vi "Bronkhorst FLOW-BUS Instrument Control Application.vi"() -> ()   [LabVIEW 2024]
doc: "This is the Control Application provided with the Bronkhorst Driver for FLOW-BUS Instruments. The application gives access to the various functions included in the driver. It can be used to test the communication and to control an instrument or as an example to get started with developing your own applications. The basic usage of the application is as follows:\n\n - Start the Application\n - Select the desired COM Port and Baud Rate\n - Click the Connect button\n\nNow data will be collected and saved (if enabled), and commands can be sent to the instrument from the various tab pages. To close the application:\n\n - Open the Setting tab\n - Click Disconnect\n - Click the Exit button to stop the application"
uses:
  <vilib>/Platform/TimedLoop/XDataNode/timing_clust.ctl
  <vilib>/Platform/TimedLoop/XDataNode/nitl_modes.ctl
  <vilib>/Platform/TimedLoop/XDataNode/wakeup.ctl
  <vilib>/Utility/error.llb/DialogType.ctl
  <vilib>/Utility/file.llb/Write To Spreadsheet File (string).vi
  <vilib>/Utility/file.llb/Write To Spreadsheet File (DBL).vi
  <vilib>/Platform/TimedLoop/XDataNode/XDataNode.xnode
  Bronkhorst FLOW-BUS.lvlib
  <vilib>/Platform/TimedLoop/XDataNode/XDNodeRunTimeDep.lvlib
panel:
  in  "Tab Control":T1(tab)=enum."Settings"
  out "Alarm Message":string
  in  "Maximum Limit":dbl=100.0 min=0.0 max=100.0 step=1.0 format="%#g%"
  in  "Minimum Limit":dbl min=0.0 max=100.0 step=1.0 format="%#g%"
  in  "Alarm setpoint mode":u32(ring) items=["No setpoint change at alarm", "Safe setpoint at alarm enabled"]
  in  "Alarm mode":u32(ring) items=["Off", "Alarm on absolute limits", "Alarm on limits related to setpoint (response alarm)", "Alarm when instrument powers up (eg. after power-down)"]
  in  "Alarm Reset Enable":T2={"Keyboard/Micro-Switch"=TRUE, "External"=TRUE, "Reset Parameter"=TRUE, "Automatic"=TRUE}
  in  "Set Alarm Settings":bool
  in  "Alarm Delay Time":u32 format="%.0f Seconds"
  in  "Alarm Setpoint":dbl min=0.0 max=100.0 step=1.0 format="%#g%"
  out "Capacity":sgl
  out "Capacity Unit Display":string
  out "Counter Value":sgl caption="Setpoint %"
  in  "Counter mode":u16(ring) items=["Off", "Counting upwards continuously", "Counting up to limit"]
  in  "Counter setpoint mode":u16(ring) items=["No setpoint change at batch limit allowed", "Setpoint change at batch limit allowed"]
  in  "Counter Setpoint":dbl min=0.0 max=100.0 step=1.0 format="%#g%"
  in  "Counter Limit":sgl min=0 max=1.001638e+07 format="%#.7f"
  in  "Counter Unit":i16(ring)=-1 items=["Select a Unit"=-1, "l"=10, "mm3"=11, "ml"=12, "cm3"=13, "ul"=14, "m3"=15, "g"=20, "mg"=21, "ug"=22, "kg"=23, "ln"=30, "mm3n"=31, "mln"=32, "cm3n"=33, "uln"=34, "dm3n"=35, "m3n"=36, "uls"=37, "mm3s"=38, "mls"=39, "cm3s"=40, "ls"=41, "dm3s"=42, "m3s"=43]
  in  "Set Counter Settings":bool
  in  "Counter Reset Enable":T2={"Keyboard/Micro-Switch"=TRUE, "External"=TRUE, "Reset Parameter"=TRUE, "Automatic"=TRUE}
  in  "Set Fluid Number":bool
  in  "Fluid Number":u8 max=7 step=1
  out "Fluid Name":string
  in  "Reset mode":u16(ring)=5 items=["No Reset", "Reset counter value (no mode change)", "Reset alarm", "Restart batch counter", "Reset counter value (counter off)", "Soft Reset"]
  in  "Reset":bool
  out "Temperature":sgl format="%#_g °C"
  out "Instrument Firmware Revision":string
  out "Analog Input Value":i16 caption="Analog Input"
  out "Instrument Modelnumber":string
  in  "Set Slope":bool
  in  "Setpoint Percentage":dbl min=0.0 max=100.0 step=1.0 format="%#.2g%"
  in  "Setpoint Direct":sgl min=0 step=1 format="%#_g mbar d"
  in  "Seconds":dbl caption="Setpoint Slope" min=0.0 max=3000.0 step=0.1 format="%#.6g Seconds"
  in  "Set Percentage":bool
  in  "Set Direct":bool
  in  "+5":bool
  in  "-5":bool
  in  "-10":bool
  in  "+10":bool
  in  "0":bool
  in  "100":bool
  in  "+1":bool
  in  "-1":bool
  in  "Wink":bool caption="Boolean"
  in  "Connect":bool
  in  "Baud Rate (38400)":u32(ring)=38400 items=["9600"=9600, "19200"=19200, "38400"=38400, "57600"=57600, "115200"=115200, "230400"=230400, "460800"=460800]
  in  "Node Address (3)":u8=3 caption="Node" min=3 max=128 step=1
  in  "Disconnect":bool
  in  "VISA resource name":refnum<visa-resource-name>
  in  "Save Data to File":bool=TRUE
  in  "Stop":bool
  in  "File Location":path
  out "Strip Chart":T3(graph)
  # "(c) 2014 Bronkhorst High-Tech B.V.  ALL RIGHTS RESERVED."
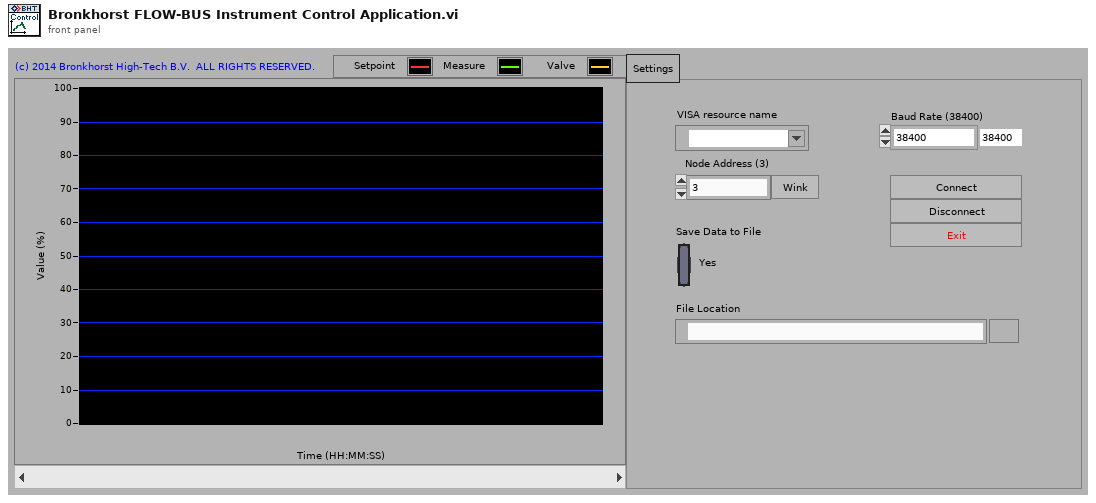
[diagram p1: front panel]
types:
  T1 = enum32{"Alarm", "Capacity", "Counter", "Fluid", "Instrument", "Setpoint", "Settings"}
  T2 = cluster{"Keyboard/Micro-Switch":bool, "External":bool, "Reset Parameter":bool, "Automatic":bool}
  T3 = cluster{"Measure Percentage":dbl, "Setpoint Percentage":dbl, "Valve Output Percentage":dbl}
  T4 = typedef "XDNodeRunTimeDep.lvlib/timing_clust.ctl" = cluster{"Expected End [f-1]":u64, "Actual End [f-1]":u64, "Finished Late? [f-1]":bool, "Expected End [i-1]":u64, "Actual End [i-1]":u64, "Finished Late? [i-1]":bool, "Expected Start [i]":u64, "Actual Start [i]":u64, "Expected Start [f]":u64, "Actual Start [f]":u64, "Source Name":string, "Structure Name":string, "Period":i64, "Deadline":i64, "Offset":i64, "Start":i64, "Priority":i32, "Timeout":i32, "Mode":T5, "Wakeup Reason":T6, "Error":errorcluster, "Source Type":string, "Secondary Source Type":string, "Global End Time":u64, "Global Start Time":u64, "Frame Duration":u64, "Iteration Duration":u64, "Assigned CPU":i32, "I/O Scan Engine Mode":u32}
  T5 = typedef "XDNodeRunTimeDep.lvlib/nitl_modes.ctl" = enum32{"No Change", "Process missed periods, maintain original phase", "Discard missed periods, maintain original phase", "Process missed periods, ignore original phase", "Discard missed periods, ignore original phase"}
  T6 = typedef "XDNodeRunTimeDep.lvlib/wakeup.ctl" = enum32{"Normal", "Aborted", "Asynchronous wakeup", "Timing source error", "Timed loop error", "Timeout"}
  T7 = enum16{"open", "replace", "create", "open or create", "replace or create", "replace or create with confirmation"}
  T8 = typedef "DialogType.ctl" = u16
  T9 = cluster{"Setpoint Percentage":dbl, "Measure Percentage":dbl, "Valve Output Percentage":dbl}
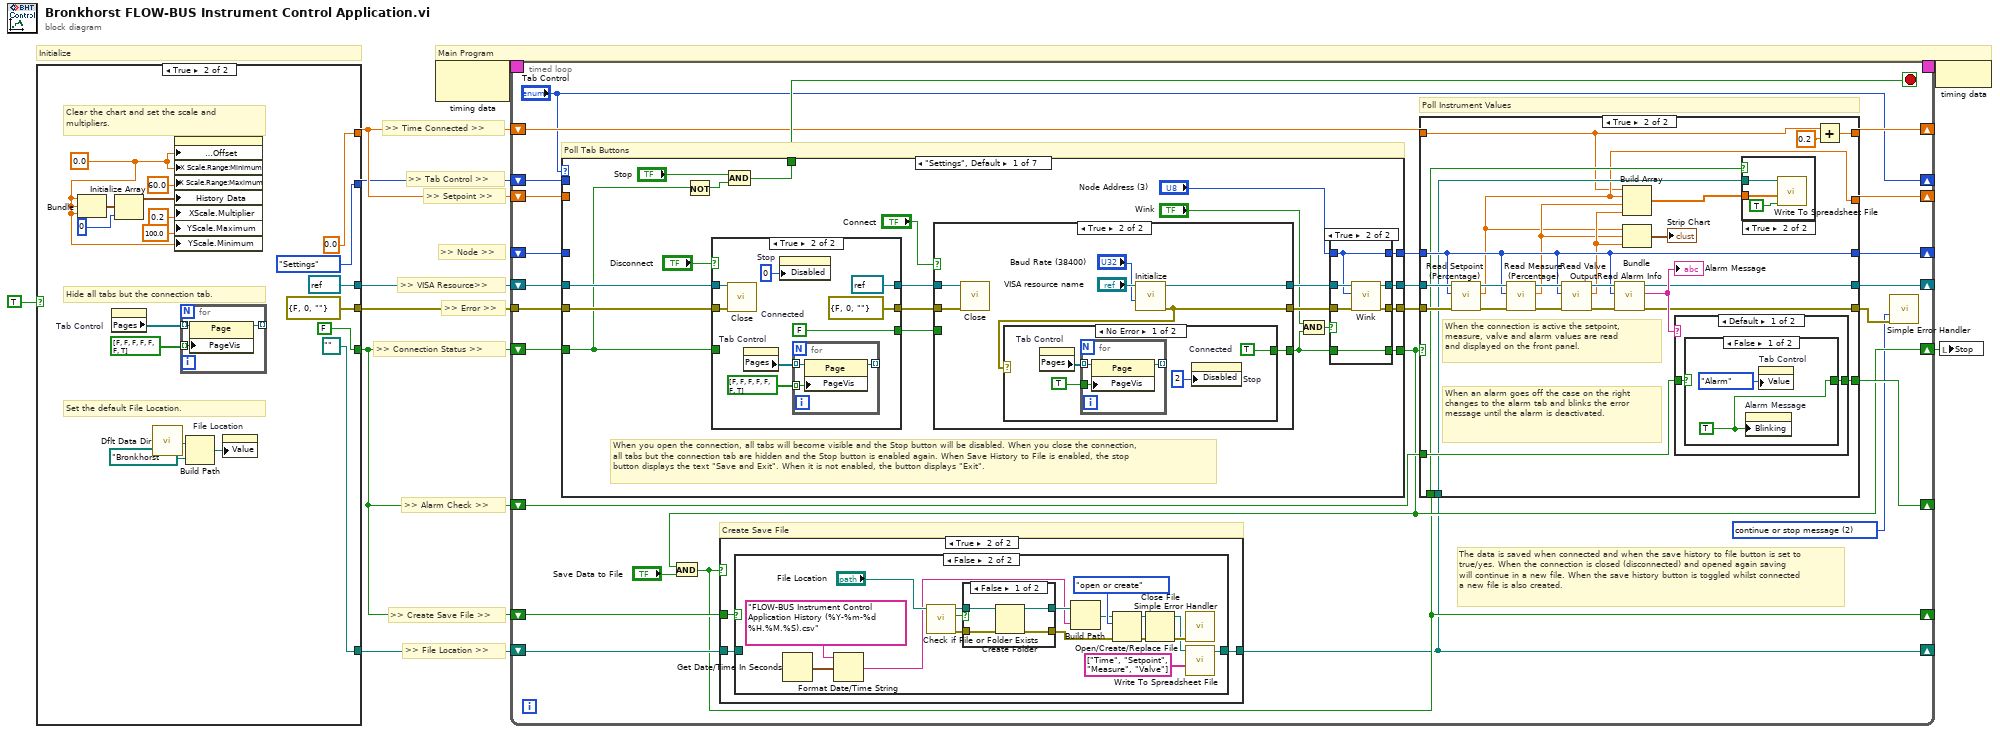
[diagram p0: block diagram]
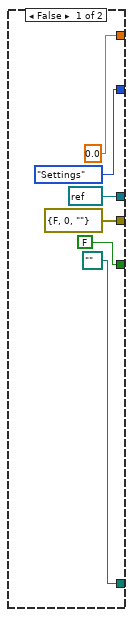
[diagram p2: hidden frame]
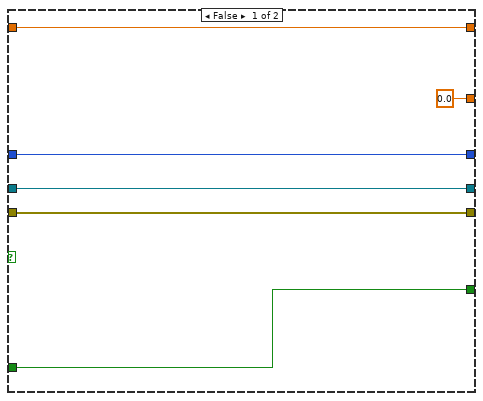
[diagram p6: hidden frame]
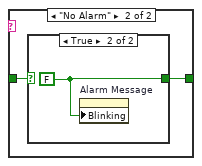
[diagram p9: hidden frame]
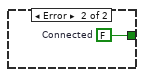
[diagram p14: hidden frame]
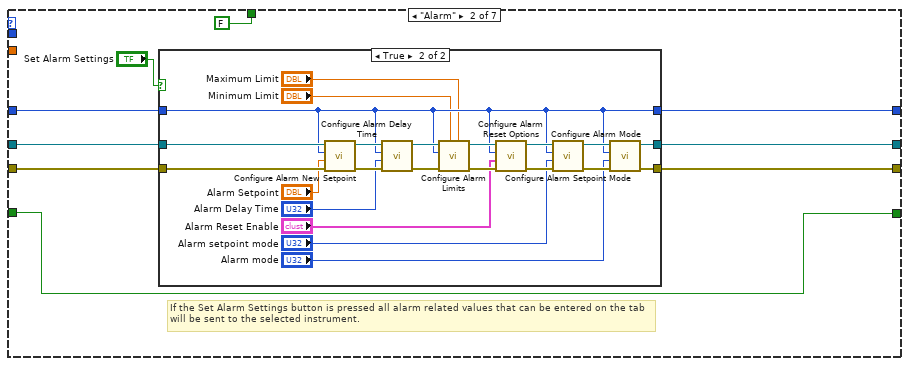
[diagram p15: hidden frame]
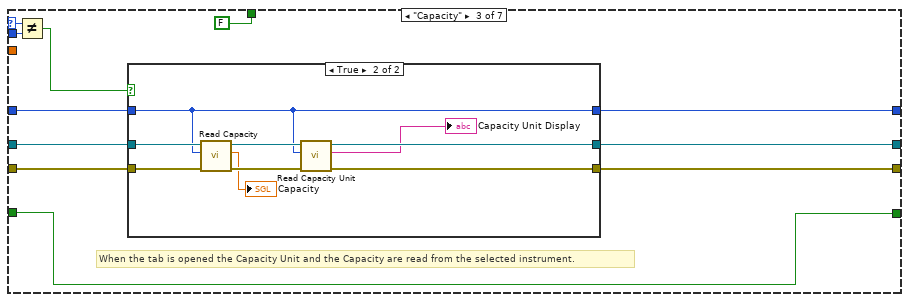
[diagram p17: hidden frame]
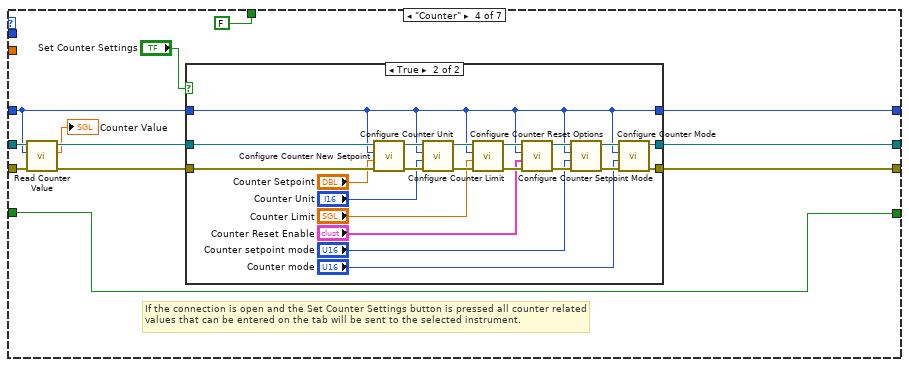
[diagram p19: hidden frame]
diagram:
  # ">> File Location >>"
  # ">> Create Save File >>"
  # "Initialize"
  # "Main Program"
  # ">> Setpoint >>"
  # ">> Time Connected >>"
  # ">> Tab Control >>"
  # ">> Alarm Check >>"
  # ">> Connection Status >>"
  # ">> Node >>"
  # ">> VISA Resource>>"
  # ">> Error >>"
  n1 = case shown="True" TRUE {
    tunnel: [errorcluster {"status"=FALSE, "code"=0, "source"=""} ("error out") errorcluster {"status"=FALSE, "code"=0, "source"=""} ("error out")] -> w1
    tunnel: [refnum<visa-resource-name> refnum ("VISA resource name out") refnum<visa-resource-name> refnum ("VISA resource name out")] -> w8
    tunnel: [T1."Settings" ("Tab Control") T1."Settings" ("Tab Control")] -> w6
    tunnel: [0.0 0.0] -> w7
    tunnel: [FALSE ("Connected") FALSE ("Connected")] -> w4
    tunnel: [path "" ("new file path (Not A Path if cancelled)") path "" ("new file path (Not A Path if cancelled)")] -> w3
    frame False {
    }
    frame True {
      w21 = 0.0
      # "Set the default File Location."
      # "Hide all tabs but the connection tab."
      # "Clear the chart and set the scale and multipliers."
      n2 = Bundle(w21, w21, w21) -> (w30:cluster{dbl, dbl, dbl})  [unwired: 1 in]
      n3 = property on="Tab Control" class="TabCtl (strict)"() -> ("Pages"=w34:refnum<vi>[])  [unwired: 2 in, 2 out]
      n4 = Initialize Array(w30, 0) -> (w32:cluster{dbl, dbl, dbl}[])
      n5 = call <vilib>:"Dflt Data Dir.vi"() -> ("App:Default Data Directory"=w18:path)
      n6 = property on="Strip Chart" class="WFChart (strict)"("X Scale.Offset and Multiplier:Offset"=w21, "X Scale.Range:Minimum"=w21, "X Scale.Range:Maximum"=60.0, "History Data"=w32, "XScale.Multiplier"=0.2 ("y"), "YScale.Maximum"=100.0, "YScale.Minimum"=w21) -> ()  [unwired: 2 in, 2 out]
      n7 = for {
        tunnel: w34 -> [w37] mode=indexing
        tunnel: bool[] [FALSE, FALSE, FALSE, FALSE, FALSE, FALSE, TRUE] -> [w36] mode=indexing
        tunnel: [w35] -> _ mode=indexing
        n8 = property class="Page"(reference=w37, "PageVis"=w36) -> (reference out=w35:refnum<vi>)  [unwired: 1 in, 1 out]
      }
      n9 = Build Path(base path=w18, name or relative path=path "Bronkhorst") -> (appended path=w20:path)
      n10 = property on="File Location" class="Path"("Value"=w20) -> ()  [unwired: 2 in, 2 out]
    }
  }
  n11 = node-c288() -> (w9:T4)  [unwired: 1 in]
  n12 = timed-loop {
    timing-out: [_] -> w10
    timing: w9 -> [_]
    shift-right: [w48] -> w2
    shift-left: w4 -> [w49]
    shift-right: [w41] -> _
    shift-left: w8 -> [w60]
    shift-right: [w42] -> _
    shift-left: _ -> [w61]
    shift-right: [w53] -> _
    shift-left: w7 -> [w62]
    shift-right: [w56] -> _
    shift-left: w4 -> [w55]
    shift-right: ["Tab Control"] -> _
    shift-left: w6 -> [w54]
    shift-right: [w52] -> _
    shift-left: w7 -> [w44]
    shift-right: [w46] -> _
    shift-left: w4 -> [w51]
    shift-right: [w45] -> _
    shift-left: w3 -> [w50]
    tunnel: w1 -> [w39]
    stop <- w63 stop-if-true
    w38 = T8 2 items=["no dialog", "OK message", "continue or stop message", "OK message + warnings", "continue/stop + warnings"] ("type of dialog (OK msg:1)")
    # "Poll Instrument Values"
    # "The data is saved when connected and when the save history to file button is set to true/yes. When the connection is closed (disconnected) and opened again saving will continue in a new file. When the save history button is toggled whilst connected a new file is also created."
    # "Create Save File"
    # "Poll Tab Buttons"
    n13 = case shown="\"Settings\", Default" "Tab Control" {
      selector: "Tab Control" -> [_ _ w237 _ w304 w333 w373]
      tunnel: [w142 w205 w234 w260 w300 w338 w369] -> w58
      tunnel: [w141 w204 w233 w261 w299 w336 w368] -> w57
      tunnel: w60 -> [w153 w203 w239 w256 w302 w328 w372]
      tunnel: w39 -> [w151 w202 w241 w259 w301 w327 w371]
      tunnel: [w136 w200 w232 w263 w296 w341 w370] -> w59
      tunnel: w61 -> [_ w201 w240 w255 w303 w326 w365]
      tunnel: [w137 w197 w235 w265 w291 w335 w375] -> w48
      tunnel: w49 -> [w144 w197 w235 w265 w291 w335 w375]
      tunnel: w62 -> [_ _ _ _ _ _ w367]
      tunnel: w54 -> [_ _ w238 _ w305 w334 w374]
      tunnel: [w146 FALSE ("stop") FALSE ("stop") FALSE ("stop") FALSE ("stop") FALSE ("stop") FALSE ("stop")] -> w63
      frame "Settings", Default {
        # "When you open the connection, all tabs will become visible and the Stop button will be disabled. When you close the connection, all tabs but the connection tab are hidden and the Stop button is enabled again. When Save History to File is enabled, the stop button displays the text \"Save and Exit\". When it is not enabled, the button displays \"Exit\"."
        n14 = Not(x=w144) -> (.not. x?=w147:bool)
        n15 = case shown="True" "Disconnect" {
          tunnel: w153 -> [w167 w172]
          tunnel: [w167 refnum<visa-resource-name> refnum ("VISA resource name out")] -> w152
          tunnel: [w166 errorcluster {"status"=FALSE, "code"=0, "source"=""} ("error out")] -> w150
          tunnel: w151 -> [w166 w171]
          tunnel: [w165 w175] -> w148
          tunnel: w144 -> [w165 _]
          frame False {
          }
          frame True {
            w175 = FALSE  # Connected
            n16 = call "Close.vi"("error in (no error)"=w171, "VISA resource name"=w172) -> ()  [unwired: 9 in, 1 out]
            n17 = property on="Tab Control" class="TabCtl (strict)"() -> ("Pages"=w173:refnum<vi>[])  [unwired: 2 in, 2 out]
            n18 = property on="Stop" class="Bool (strict)"("Disabled"=u8 0) -> ()  [unwired: 2 in, 2 out]
            n19 = for {
              tunnel: w173 -> [w178] mode=indexing
              tunnel: [w177] -> _ mode=indexing
              tunnel: bool[] [FALSE, FALSE, FALSE, FALSE, FALSE, FALSE, TRUE] -> [w176] mode=indexing
              n20 = property class="Page"(reference=w178, "PageVis"=w176) -> (reference out=w177:refnum<vi>)  [unwired: 1 in, 1 out]
            }
          }
        }
        n21 = And(x="Stop", y=w147) -> (x .and. y?=w146:bool)
        n22 = case shown="True" "Connect" {
          tunnel: [w180 w183] -> w140
          tunnel: [w181 w182] -> w139
          tunnel: w152 -> [w180 w185]
          tunnel: w150 -> [w181 w186]
          tunnel: [w179 w184] -> w134
          tunnel: w148 -> [w179 _]
          frame False {
          }
          frame True {
            n23 = call "Close.vi"("error in (no error)"=w186, "VISA resource name"=w185) -> ()  [unwired: 9 in, 1 out]
            n24 = call "Initialize.vi"("Baud Rate (38400)"="Baud Rate (38400)", "VISA resource name"="VISA resource name") -> ("error out"=w182:errorcluster, "VISA resource name out"=w183:refnum<visa-resource-name>)  [unwired: 8 in]
            n25 = case shown="No Error" w182 {
              tunnel: [w189 w196] -> w184
              frame No Error {
                w189 = TRUE  # Connected
                n26 = property on="Tab Control" class="TabCtl (strict)"() -> ("Pages"=w191:refnum<vi>[])  [unwired: 2 in, 2 out]
                n27 = for {
                  tunnel: w191 -> [w195] mode=indexing
                  tunnel: TRUE -> [w194]
                  tunnel: [w193] -> _ mode=indexing
                  n28 = property class="Page"(reference=w195, "PageVis"=w194) -> (reference out=w193:refnum<vi>)  [unwired: 1 in, 1 out]
                }
                n29 = property on="Stop" class="Bool (strict)"("Disabled"=u8 2) -> ()  [unwired: 2 in, 2 out]
              }
              frame Error {
                w196 = FALSE  # Connected
              }
            }
          }
        }
        n30 = And(x="Wink", y=w134) -> (x .and. y?=w138:bool)
        n31 = case shown="True" w138 {
          tunnel: "Node Address (3)" -> [w155 w159]
          tunnel: [w158 w164] -> w142
          tunnel: [w157 w163] -> w141
          tunnel: w140 -> [w158 w161]
          tunnel: w139 -> [w157 w162]
          tunnel: [w156 w160] -> w137
          tunnel: w134 -> [w156 w160]
          tunnel: [w155 w159] -> w136
          frame False {
          }
          frame True {
            n32 = call "Wink.vi"("error in (no error)"=w162, "Node (3)"=w159, "VISA resource name"=w161) -> ("error out"=w163:errorcluster, "VISA resource name out"=w164:refnum<visa-resource-name>)  [unwired: 7 in]
          }
        }
      }
      frame "Alarm" {
        # "If the Set Alarm Settings button is pressed all alarm related values that can be entered on the tab will be sent to the selected instrument."
        n33 = case shown="True" "Set Alarm Settings" {
          tunnel: w203 -> [w207 w230]
          tunnel: w202 -> [w206 w229]
          tunnel: w201 -> [w208 w213]
          tunnel: [w207 w223] -> w205
          tunnel: [w206 w222] -> w204
          tunnel: [w208 w213] -> w200
          frame False {
          }
          frame True {
            n34 = call "Configure Alarm New Setpoint.vi"("error in (no error)"=w229, "Alarm Setpoint (0%)"="Alarm Setpoint", "Node (3)"=w213, "VISA resource name"=w230) -> ("error out"=w227:errorcluster, "VISA resource name out"=w228:refnum<visa-resource-name>)  [unwired: 6 in]
            n35 = call "Configure Alarm Delay Time.vi"("error in (no error)"=w227, "Alarm Delay Time (0 Seconds)"="Alarm Delay Time", "Node (3)"=w213, "VISA resource name"=w228) -> ("error out"=w214:errorcluster, "VISA resource name out"=w217:refnum<visa-resource-name>)  [unwired: 6 in]
            n36 = call "Configure Alarm Limits.vi"("Maximum Limit (100%)"="Maximum Limit", "Minimum Limit (0%)"="Minimum Limit", "error in (no error)"=w214, "Node (3)"=w213, "VISA resource name"=w217) -> ("error out"=w215:errorcluster, "VISA resource name out"=w216:refnum<visa-resource-name>)  [unwired: 5 in]
            n37 = call "Configure Alarm Reset Options.vi"("error in (no error)"=w215, "Alarm Reset (All Enabled)"="Alarm Reset Enable", "Node (3)"=w213, "VISA resource name"=w216) -> ("error out"=w224:errorcluster, "VISA resource name out"=w225:refnum<visa-resource-name>)  [unwired: 6 in]
            n38 = call "Configure Alarm Setpoint Mode.vi"("error in (no error)"=w224, "Alarm Setpoint Mode (0: No setpoint)"="Alarm setpoint mode", "Node (3)"=w213, "VISA resource name"=w225) -> ("error out"=w221:errorcluster, "VISA resource name out"=w220:refnum<visa-resource-name>)  [unwired: 6 in]
            n39 = call "Configure Alarm Mode.vi"("error in (no error)"=w221, "Alarm mode (0: Off)"="Alarm mode", "Node (3)"=w213, "VISA resource name"=w220) -> ("error out"=w222:errorcluster, "VISA resource name out"=w223:refnum<visa-resource-name>)  [unwired: 6 in]
          }
        }
      }
      frame "Capacity" {
        # "When the tab is opened the Capacity Unit and the Capacity are read from the selected instrument."
        n40 = Not Equal?(x=w237, y=w238) -> (x != y?=w231:bool)
        n41 = case shown="True" w231 {
          tunnel: w239 -> [w243 w253]
          tunnel: w241 -> [w242 w252]
          tunnel: w240 -> [w244 w246]
          tunnel: [w243 w248] -> w234
          tunnel: [w242 w249] -> w233
          tunnel: [w244 w246] -> w232
          frame False {
          }
          frame True {
            n42 = call "Read Capacity.vi"("error in (no error)"=w252, "Node (3)"=w246, "VISA resource name"=w253) -> ("error out"=w250:errorcluster, "Capacity"=→"Capacity":sgl, "VISA resource name out"=w251:refnum<visa-resource-name>)  [unwired: 6 in]
            n43 = call "Read Capacity Unit.vi"("error in (no error)"=w250, "Node (3)"=w246, "VISA resource name"=w251) -> ("error out"=w249:errorcluster, "Capacity Unit"=→"Capacity Unit Display":string, "VISA resource name out"=w248:refnum<visa-resource-name>)  [unwired: 6 in]
          }
        }
      }
      frame "Counter" {
        # "If the connection is open and the Set Counter Settings button is pressed all counter related values that can be entered on the tab will be sent to the selected instrument."
        n44 = call "Read Counter Value.vi"("error in (no error)"=w259, "Node (3)"=w255, "VISA resource name"=w256) -> ("error out"=w258:errorcluster, "Counter Value"=→"Counter Value":sgl, "VISA resource name out"=w257:refnum<visa-resource-name>)  [unwired: 6 in]
        n45 = case shown="True" "Set Counter Settings" {
          tunnel: w257 -> [w267 w274]
          tunnel: w258 -> [w266 w273]
          tunnel: w255 -> [w268 w269]
          tunnel: [w267 w272] -> w260
          tunnel: [w266 w271] -> w261
          tunnel: [w268 w269] -> w263
          frame False {
          }
          frame True {
            n46 = call "Configure Counter New Setpoint.vi"("error in (no error)"=w273, "Counter Setpoint (0%)"="Counter Setpoint", "Node (3)"=w269, "VISA resource name"=w274) -> ("error out"=w280:errorcluster, "VISA resource name out"=w289:refnum<visa-resource-name>)  [unwired: 6 in]
            n47 = call "Configure Counter Unit.vi"("error in (no error)"=w280, "Counter Unit (-1:Select a Unit)"="Counter Unit", "Node (3)"=w269, "VISA resource name"=w289) -> ("error out"=w281:errorcluster, "VISA resource name out"=w288:refnum<visa-resource-name>)  [unwired: 6 in]
            n48 = call "Configure Counter Limit.vi"("error in (no error)"=w281, "Counter Limit (0)"="Counter Limit", "Node (3)"=w269, "VISA resource name"=w288) -> ("error out"=w282:errorcluster, "VISA resource name out"=w287:refnum<visa-resource-name>)  [unwired: 6 in]
            n49 = call "Configure Counter Reset Options.vi"("error in (no error)"=w282, "Counter Reset (All Enabled)"="Counter Reset Enable", "Node (3)"=w269, "VISA resource name"=w287) -> ("error out"=w283:errorcluster, "VISA resource name out"=w286:refnum<visa-resource-name>)  [unwired: 6 in]
            n50 = call "Configure Counter Setpoint Mode.vi"("error in (no error)"=w283, "Counter setpoint mode (0: No setpoint change)"="Counter setpoint mode", "Node (3)"=w269, "VISA resource name"=w286) -> ("error out"=w284:errorcluster, "VISA resource name out"=w285:refnum<visa-resource-name>)  [unwired: 6 in]
            n51 = call "Configure Counter Mode.vi"("error in (no error)"=w284, "Counter Mode (0: Off)"="Counter mode", "Node (3)"=w269, "VISA resource name"=w285) -> ("error out"=w271:errorcluster, "VISA resource name out"=w272:refnum<visa-resource-name>)  [unwired: 6 in]
          }
        }
      }
      frame "Fluid" {
        # "If the connection is open and the Set Fluid Number button is pressed, the selected fluid number will be sent to, and the fluid name will be read from the selected instrument. When the tab is opened the Fluid name will be read from the selected instrument."
        n52 = Not Equal?(x=w304, y=w305) -> (x != y?=w292:bool)
        n53 = case shown="True" "Set Fluid Number" {
          tunnel: [w317 w319] -> w295
          tunnel: w303 -> [w317 w319]
          tunnel: w302 -> [w316 w323]
          tunnel: w301 -> [w315 w322]
          tunnel: [w316 w321] -> w297
          tunnel: [w315 w320] -> w298
          frame False {
          }
          frame True {
            n54 = call "Configure Fluid Number.vi"("error in (no error)"=w322, "Fluid Number (0)"="Fluid Number", "Node (3)"=w319, "VISA resource name"=w323) -> ("error out"=w320:errorcluster, "VISA resource name out"=w321:refnum<visa-resource-name>)  [unwired: 6 in]
          }
        }
        n55 = Or(x=w292, y="Set Fluid Number") -> (x .or. y?=w294:bool)
        n56 = case shown="True" w294 {
          tunnel: [w307 w314] -> w300
          tunnel: [w306 w313] -> w299
          tunnel: w298 -> [w306 w312]
          tunnel: w297 -> [w307 w311]
          tunnel: [w308 w310] -> w296
          tunnel: w295 -> [w308 w310]
          frame False {
          }
          frame True {
            n57 = call "Read Fluid Name.vi"("error in (no error)"=w312, "Node (3)"=w310, "VISA resource name"=w311) -> ("error out"=w313:errorcluster, "Fluid Name"=→"Fluid Name":string, "VISA resource name out"=w314:refnum<visa-resource-name>)  [unwired: 6 in]
          }
        }
      }
      frame "Instrument" {
        # "When the tab is opened, all values on the tab will be read from the selected instrument. When the connection is active and the reset button is pressed, the selected reset command will be sent to the selected instrument."
        n58 = Not Equal?(x=w333, y=w334) -> (x != y?=w332:bool)
        n59 = call "Read Analog Input.vi"("error in (no error)"=w327, "Node (3)"=w326, "VISA resource name"=w328) -> ("error out"=w330:errorcluster, "Analog Input Value"=→"Analog Input Value":i16, "VISA resource name out"=w329:refnum<visa-resource-name>)  [unwired: 6 in]
        n60 = case shown="True" w332 {
          tunnel: w329 -> [w352 w359]
          tunnel: w330 -> [w351 w360]
          tunnel: w326 -> [w353 w357]
          tunnel: [w352 w363] -> w339
          tunnel: [w351 w362] -> w337
          tunnel: [w353 w357] -> w340
          frame False {
          }
          frame True {
            n61 = call "Read Temperature.vi"("error in (no error)"=w360, "Node (3)"=w357, "VISA resource name"=w359) -> ("error out"=w356:errorcluster, "Temperature (deg C)"=→"Temperature":sgl, "VISA resource name out"=w355:refnum<visa-resource-name>)  [unwired: 6 in]
            n62 = call "Revision Query.vi"("error in (no error)"=w356, "Node (3)"=w357, "VISA resource name"=w355) -> ("error out"=w362:errorcluster, "Instrument Firmware Revision"=→"Instrument Firmware Revision":string, "VISA resource name out"=w363:refnum<visa-resource-name>, "Instrument Modelnumber"=→"Instrument Modelnumber":string)  [unwired: 4 in, 1 out]
          }
        }
        n63 = case shown="True" "Reset" {
          tunnel: w340 -> [w344 w348]
          tunnel: [w344 w348] -> w341
          tunnel: w339 -> [w343 w350]
          tunnel: [w343 w346] -> w338
          tunnel: [w342 w345] -> w336
          tunnel: w337 -> [w342 w349]
          frame False {
          }
          frame True {
            n64 = call "Reset.vi"("error in (no error)"=w349, "Reset mode (5: Soft Reset)"="Reset mode", "Node (3)"=w348, "VISA resource name"=w350) -> ("error out"=w345:errorcluster, "VISA resource name out"=w346:refnum<visa-resource-name>)  [unwired: 6 in]
          }
        }
      }
      frame "Setpoint" {
        # "When the tab is opened the setpoint is read from the instrument (both percentage and direct) and displayed in the indicators. When any of the buttons are pressed the corresponding action is performed."
        n65 = Not Equal?(x=w373, y=w374) -> (x != y?=w364:bool)
        n66 = case shown="True" w364 {
          tunnel: [w390 w504] -> w370
          tunnel: w365 -> [w395 w504]
          tunnel: w372 -> [w393 w511]
          tunnel: w371 -> [w394 w510]
          tunnel: [w389 w502] -> w368
          tunnel: [w392 w503] -> w369
          tunnel: w367 -> [w391 _]
          frame False {
            # "The booleans are turned into a number so multiple buttons can be checked in one case."
            n67 = Build Array("-5", "+5", "-10", "+10", "0", "100", "-1", "+1") -> (w384:bool[])
            n68 = Boolean Array To Number(Boolean array=w384) -> (number=w388:u32)
            n69 = case shown="1" w388 {
              tunnel: [w408 w421 w429 w437 w443 w449 w457 w465 w470] -> w405
              tunnel: w395 -> [w408 w421 w429 w437 w443 w449 w457 w465 w470]
              tunnel: [w415 w423 w431 w439 w445 w451 w459 w467 w469] -> w406
              tunnel: w393 -> [w413 w420 w428 w436 w442 w448 w456 w464 w469]
              tunnel: w394 -> [w412 w419 w427 w435 w441 w447 w455 w463 w468]
              tunnel: [w414 w422 w430 w438 w444 w450 w458 w466 w468] -> w407
              tunnel: w391 -> [w410 w417 w425 w433 _ _ w453 w461 _]
              frame 1 {
                n70 = Subtract(x=w410, y=5.0) -> (x-y=w409:dbl)
                n71 = call "Configure Setpoint (Percentage).vi"("error in (no error)"=w412, "Setpoint Percentage (0%)"=w409, "Node (3)"=w408, "VISA resource name"=w413) -> ("error out"=w414:errorcluster, "VISA resource name out"=w415:refnum<visa-resource-name>)  [unwired: 6 in]
              }
              frame 2 {
                n72 = Add(x=w417, y=5.0) -> (x+y=w416:dbl)
                n73 = call "Configure Setpoint (Percentage).vi"("error in (no error)"=w419, "Setpoint Percentage (0%)"=w416, "Node (3)"=w421, "VISA resource name"=w420) -> ("error out"=w422:errorcluster, "VISA resource name out"=w423:refnum<visa-resource-name>)  [unwired: 6 in]
              }
              frame 4 {
                n74 = Subtract(x=w425, y=10.0) -> (x-y=w424:dbl)
                n75 = call "Configure Setpoint (Percentage).vi"("error in (no error)"=w427, "Setpoint Percentage (0%)"=w424, "Node (3)"=w429, "VISA resource name"=w428) -> ("error out"=w430:errorcluster, "VISA resource name out"=w431:refnum<visa-resource-name>)  [unwired: 6 in]
              }
              frame 8 {
                n76 = Add(x=w433, y=10.0) -> (x+y=w432:dbl)
                n77 = call "Configure Setpoint (Percentage).vi"("error in (no error)"=w435, "Setpoint Percentage (0%)"=w432, "Node (3)"=w437, "VISA resource name"=w436) -> ("error out"=w438:errorcluster, "VISA resource name out"=w439:refnum<visa-resource-name>)  [unwired: 6 in]
              }
              frame 16 {
                n78 = call "Configure Setpoint (Percentage).vi"("error in (no error)"=w441, "Setpoint Percentage (0%)"=0.0 ("y"), "Node (3)"=w443, "VISA resource name"=w442) -> ("error out"=w444:errorcluster, "VISA resource name out"=w445:refnum<visa-resource-name>)  [unwired: 6 in]
              }
              frame 32 {
                n79 = call "Configure Setpoint (Percentage).vi"("error in (no error)"=w447, "Setpoint Percentage (0%)"=100.0 ("y"), "Node (3)"=w449, "VISA resource name"=w448) -> ("error out"=w450:errorcluster, "VISA resource name out"=w451:refnum<visa-resource-name>)  [unwired: 6 in]
              }
              frame 64 {
                n80 = Subtract(x=w453, y=1.0) -> (x-y=w452:dbl)
                n81 = call "Configure Setpoint (Percentage).vi"("error in (no error)"=w455, "Setpoint Percentage (0%)"=w452, "Node (3)"=w457, "VISA resource name"=w456) -> ("error out"=w458:errorcluster, "VISA resource name out"=w459:refnum<visa-resource-name>)  [unwired: 6 in]
              }
              frame 128 {
                n82 = Add(x=w461, y=1.0) -> (x+y=w460:dbl)
                n83 = call "Configure Setpoint (Percentage).vi"("error in (no error)"=w463, "Setpoint Percentage (0%)"=w460, "Node (3)"=w465, "VISA resource name"=w464) -> ("error out"=w466:errorcluster, "VISA resource name out"=w467:refnum<visa-resource-name>)  [unwired: 6 in]
              }
              frame Default {
              }
            }
            n84 = case shown="True" "Set Slope" {
              tunnel: [w471 w474] -> w400
              tunnel: [w472 w475] -> w401
              tunnel: [w473 w478] -> w403
              tunnel: w405 -> [w473 w478]
              tunnel: w407 -> [w472 w477]
              tunnel: "Seconds" -> [_ w476]
              tunnel: w406 -> [w471 w479]
              frame False {
              }
              frame True {
                n85 = call "Configure Setpoint Slope.vi"("error in (no error)"=w477, "Setpoint Slope (0 Seconds)"=w476, "Node (3)"=w478, "VISA resource name"=w479) -> ("error out"=w475:errorcluster, "VISA resource name out"=w474:refnum<visa-resource-name>)  [unwired: 6 in]
              }
            }
            n86 = case shown="True" "Set Percentage" {
              tunnel: [w491 w495] -> w399
              tunnel: [w490 w494] -> w398
              tunnel: w400 -> [w491 w497]
              tunnel: w401 -> [w490 w496]
              tunnel: "Setpoint Percentage" -> [_ w492]
              tunnel: w403 -> [w489 w493]
              tunnel: [w489 w493] -> w404
              frame False {
              }
              frame True {
                n87 = call "Configure Setpoint (Percentage).vi"("error in (no error)"=w496, "Setpoint Percentage (0%)"=w492, "Node (3)"=w493, "VISA resource name"=w497) -> ("error out"=w494:errorcluster, "VISA resource name out"=w495:refnum<visa-resource-name>)  [unwired: 6 in]
              }
            }
            n88 = case shown="True" "Set Direct" {
              tunnel: [w481 w486] -> w392
              tunnel: [w482 w485] -> w389
              tunnel: w399 -> [w481 w488]
              tunnel: w398 -> [w482 w487]
              tunnel: "Setpoint Direct" -> [_ w484]
              tunnel: [w480 w483] -> w390
              tunnel: w404 -> [w480 w483]
              frame False {
              }
              frame True {
                n89 = call "Configure Setpoint (Direct).vi"("error in (no error)"=w487, "Setpoint Direct (0)"=w484, "Node (3)"=w483, "VISA resource name"=w488) -> ("error out"=w485:errorcluster, "VISA resource name out"=w486:refnum<visa-resource-name>)  [unwired: 6 in]
              }
            }
          }
          frame True {
            n90 = call "Read Setpoint (Percentage).vi"("error in (no error)"=w510, "Node (3)"=w504, "VISA resource name"=w511) -> ("error out"=w508:errorcluster, "Setpoint Percentage"=w507:dbl, "VISA resource name out"=w509:refnum<visa-resource-name>)  [unwired: 6 in]
            n91 = call "Read Setpoint (Direct).vi"("error in (no error)"=w508, "Node (3)"=w504, "VISA resource name"=w509) -> ("error out"=w506:errorcluster, "Setpoint Direct"=w498:sgl, "VISA resource name out"=w505:refnum<visa-resource-name>)  [unwired: 6 in]
            n92 = call "Read Capacity Unit.vi"("error in (no error)"=w506, "Node (3)"=w504, "VISA resource name"=w505) -> ("error out"=w502:errorcluster, "Capacity Unit"=w499:string, "VISA resource name out"=w503:refnum<visa-resource-name>)  [unwired: 6 in]
            n93 = Concatenate Strings("%#_g ", w499) -> (w501:string)
            n94 = local write "Setpoint Direct"(w498) -> ()
            n95 = local write "Setpoint Percentage"(w507) -> ()
            n96 = property on="Setpoint Direct" class="DigNum (strict)"("FormatString"=w501) -> ()  [unwired: 2 in, 2 out]
          }
        }
      }
    }
    n97 = And(x=w48, y="Save Data to File") -> (x .and. y?=w46:bool)
    n98 = case shown="True" w46 {
      tunnel: [w64 w67] -> w45
      tunnel: w51 -> [_ w66]
      tunnel: w50 -> [w64 w65]
      frame False {
      }
      frame True {
        n99 = case shown="False" w66 {
          tunnel: [w68 w71] -> w67
          tunnel: w65 -> [w68 _]
          frame True {
          }
          frame False {
            n100 = Get Date/Time In Seconds() -> (seconds since 1Jan1904=w73:timestamp)
            n101 = Format Date/Time String(time format string (%c)="FLOW-BUS Instrument Control Application History (%Y-%m-%d %H.%M.%S).csv", seconds (now)=w73) -> (date/time string=w69:string)  [unwired: 1 in]
            n102 = call <vilib>:"Check if File or Folder Exists.vi"("path"="File Location") -> ("error out"=w79:errorcluster, "file or folder exists?"=w77:bool, "dup path"=w78:path)  [unwired: 8 in]
            n103 = case shown="False" w77 {
              tunnel: w78 -> [w89 w91]
              tunnel: w79 -> [w88 w90]
              tunnel: [w87 w91] -> w80
              tunnel: [w86 w90] -> w75
              frame False {
                n104 = Create Folder(path (use dialog)=w89, error in=w88) -> (created path=w87:path, error out=w86:errorcluster)  [unwired: 1 in, 1 out]
              }
              frame True {
              }
            }
            n105 = Build Path(base path=w80, name or relative path=w69) -> (appended path=w76:path)
            n106 = Open/Create/Replace File(file path (use dialog)=w76, error in=w75, operation (0:open)=T7."open or create") -> (refnum out=w84:refnum<file>, error out=w85:errorcluster)  [unwired: 3 in, 1 out]
            n107 = Close File(refnum=w84, error in=w85) -> (path=w72:path, error out=w82:errorcluster)
            n108 = call <vilib>:"Simple Error Handler.vi"("error in (no error)"=w82) -> ()  [unwired: 4 in, 5 out]
            n109 = call-poly <vilib>:"Write To Spreadsheet File.vi"("1D data"=string[] ["Time", "Setpoint", "Measure", "Valve"], "file path (dialog if empty)"=w72) -> ("new file path (Not A Path if cancelled)"=w71:path)  [unwired: 6 in]
          }
        }
      }
    }
    n110 = case shown="True" w48 {
      tunnel: w57 -> [w96 w117]
      tunnel: w58 -> [w97 w116]
      tunnel: [w96 w107] -> w40
      tunnel: [w97 w108] -> w41
      tunnel: w59 -> [w95 w113]
      tunnel: [w95 w113] -> w42
      tunnel: [0.0 ("y") w100] -> w53
      tunnel: [w94 w111] -> w56
      tunnel: w55 -> [w94 w110]
      tunnel: w44 -> [w93 w98]
      tunnel: [w93 w101] -> w52
      tunnel: w45 -> [_ w103]
      tunnel: w46 -> [_ w102]
      frame False {
      }
      frame True {
        # "When the connection is active the setpoint,\nmeasure, valve and alarm values are read \nand displayed on the front panel."
        # "When an alarm goes off the case on the right changes to the alarm tab and blinks the error message until the alarm is deactivated."
        n111 = call "Read Setpoint (Percentage).vi"("error in (no error)"=w117, "Node (3)"=w113, "VISA resource name"=w116) -> ("error out"=w118:errorcluster, "Setpoint Percentage"=w100:dbl, "VISA resource name out"=w119:refnum<visa-resource-name>)  [unwired: 6 in]
        n112 = call "Read Measure (Percentage).vi"("error in (no error)"=w118, "Node (3)"=w113, "VISA resource name"=w119) -> ("error out"=w120:errorcluster, "Measure Percentage"=w104:dbl, "VISA resource name out"=w121:refnum<visa-resource-name>)  [unwired: 6 in]
        n113 = call "Read Valve Output.vi"("error in (no error)"=w120, "Node (3)"=w113, "VISA resource name"=w121) -> ("error out"=w114:errorcluster, "Valve Output Percentage"=w105:dbl, "VISA resource name out"=w115:refnum<visa-resource-name>)  [unwired: 5 in, 1 out]
        n114 = call "Read Alarm Info.vi"("error in (no error)"=w114, "Node (3)"=w113, "VISA resource name"=w115) -> ("error out"=w107:errorcluster, "Alarm Message"=w112:string, "VISA resource name out"=w108:refnum<visa-resource-name>)  [unwired: 6 in]
        "Alarm Message" <- w112
        n115 = Build Array(w98, w100, w104, w105) -> (w99:dbl[])
        n116 = Bundle("Setpoint Percentage"=w100, "Measure Percentage"=w104, "Valve Output Percentage"=w105) -> (→"Strip Chart":T9)  [unwired: 1 in]
        n117 = case shown="Default" w112 {
          tunnel: w110 -> [w126 w130]
          tunnel: [w125 w131] -> w111
          frame Default {
            n118 = case shown="False" w126 {
              selector: w126 -> [_ w129]
              tunnel: [w127 w129] -> w125
              frame False {
                w127 = TRUE
                n119 = property on="Alarm Message" class="Str"("Blinking"=w127) -> ()  [unwired: 2 in, 2 out]
                n120 = property on="Tab Control" class="TabCtl (strict)"("Value"=T1."Alarm" ("Tab Control")) -> ()  [unwired: 2 in, 2 out]
              }
              frame True {
              }
            }
          }
          frame "No Alarm" {
            n121 = case shown="True" w130 {
              selector: w130 -> [w132 _]
              tunnel: [w132 w133] -> w131
              frame False {
              }
              frame True {
                w133 = FALSE ("Blinking")
                n122 = property on="Alarm Message" class="Str"("Blinking"=w133) -> ()  [unwired: 2 in, 2 out]
              }
            }
          }
        }
        n123 = case shown="True" w102 {
          tunnel: w99 -> [_ w123]
          tunnel: w103 -> [_ w122]
          frame False {
          }
          frame True {
            n124 = call-poly <vilib>:"Write To Spreadsheet File.vi"("append to file? (new file:F)"=TRUE, "1D data"=w123, "file path (dialog if empty)"=w122) -> ()  [unwired: 5 in, 1 out]
          }
        }
        n125 = Add(x=w98, y=0.2) -> (x+y=w101:dbl)
      }
    }
    n126 = call <vilib>:"Simple Error Handler.vi"("type of dialog (OK msg:1)"=w38, "error in (no error)"=w40) -> ()  [unwired: 3 in, 5 out]
  }
  n127 = node-c288(w10) -> ()
  n128 = local write "Stop"(w2) -> ()
